vi "shoot.vi"(1 "Shooting Activated":bool, 8 "error in (no error)":errorcluster, 10 "Motor Power":dbl, 11 "refnum name":string="My Motor RefNum") -> (0 "error out":errorcluster)   [LabVIEW 2016, in "External.lvlib"]
uses:
  External.lvlib
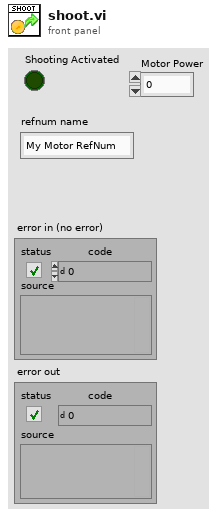
[diagram p1: front panel]
types:
  T1 = typedef "WPI_MotorControlDeviceRef.ctl" = cluster{"DeviceStatus":errorcluster, "Type":T2, "PWM":cluster{"PWM Channel":T3, "DeadBand":T4}, "CAN":cluster{"Device Number":u8, "SetOutput VI Ref":variant, "GetOutput VI Ref":variant, "Enable VI Ref":variant, "Disable VI Ref":variant, "Data":variant}, "Invert":bool}
  T2 = typedef "WPI_MotorControlType.ctl" = enum16{"PWM", "CAN"}
  T3 = typedef "FPGA_DIOPWMChannel.ctl" = enum8{"PWM 0", "PWM 1", "PWM 2", "PWM 3", "PWM 4", "PWM 5", "PWM 6", "PWM 7", "PWM 8", "PWM 9", "PWM MXP 0", "PWM MXP 1", "PWM MXP 2", "PWM MXP 3", "PWM MXP 4", "PWM MXP 5", "PWM MXP 6", "PWM MXP 7", "PWM MXP 8", "PWM MXP 9", "Invalid"}
  T4 = typedef "WPI_PWMDeadband.ctl" = cluster{"Name":string, "maxPositivePwm":i32, "minPositivePwm":i32, "centerPwm":i32, "maxNegativePwm":i32, "minNegativePwm":i32, "angularRange":u16}
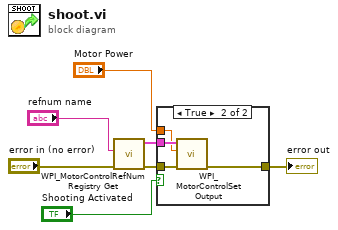
[diagram p0: block diagram]
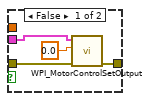
[diagram p2: hidden frame]
diagram:
  n1 = call <vilib>:"WPI_MotorControlRefNum Registry Get.vi"("error in (no error)"="error in (no error)", "refnum name"="refnum name") -> ("error out"=w5:errorcluster, "MotorControlDevRef"=w6:T1)  [unwired: 8 in]
  n2 = case shown="True" "Shooting Activated" {
    tunnel: w6 -> [w11 w15]
    tunnel: w5 -> [w10 w14]
    tunnel: "Motor Power" -> [_ w13]
    tunnel: [w8 w12] -> w2
    frame False {
      n3 = call <vilib>:"WPI_MotorControlSetOutput.vi"("error in (no error)"=w10, "Output"=0.0, "MotorControlDevRef"=w11) -> ("error out"=w8:errorcluster)  [unwired: 6 in, 2 out]
    }
    frame True {
      n4 = call <vilib>:"WPI_MotorControlSetOutput.vi"("error in (no error)"=w14, "Output"=w13, "MotorControlDevRef"=w15) -> ("error out"=w12:errorcluster)  [unwired: 6 in, 2 out]
    }
  }
  "error out" <- w2
